vi "decodeStream.vi"(8 "error in (no error)":errorcluster, 9 "beginIndex":i32, 10 "binary stream":u8[](array[numeric]), 11 "tBSONBinary in":refnum<class "tBSONBinary.lvclass">) -> (0 "error out":errorcluster, 1 "endIndex":i32, 2 "binary stream out":u8[](array[numeric]), 3 "tBSONBinary out":refnum<class "tBSONBinary.lvclass">)   [LabVIEW 2013, in "BSON.lvlib" / "tBSONBinary.lvclass"]
uses:
  tBSONBinary.lvclass
  tBSONElement/tBSONElement.lvclass
  status.ctl
  Subtype.ctl
  setSubtype.vi
  setValue.vi
  BSON.lvlib
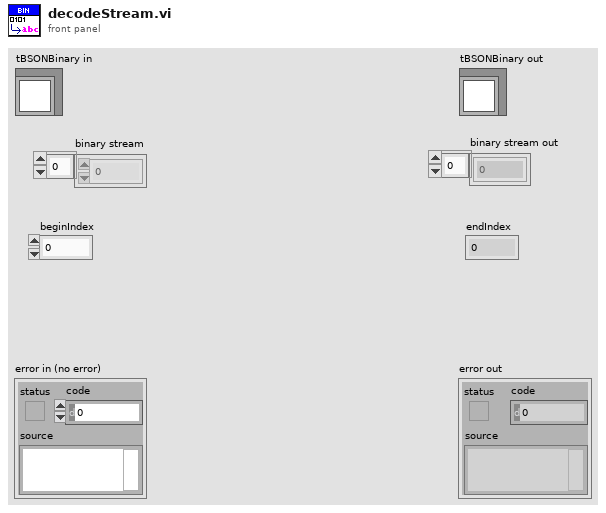
[diagram p1: front panel]
types:
  T1 = typedef "BSON.lvlib/status.ctl" = enum16{"Stream Corrupted or Ended Abruptly", "Incorrect Type In Stream", "ObjectID Invalid", "Method Not Implemented", "Invalid Name", "Invalid URI", "AutoReconnect", "Operation Failed", "Incorrectly Configured", "Cursor Not Found", "Timeout", "Invalid Type", "Empty Name", "Duplicate Name", "MD5Incorrect"}
  T2 = typedef "BSON.lvlib/tBSONBinary.lvclass/Subtype.ctl" = u8
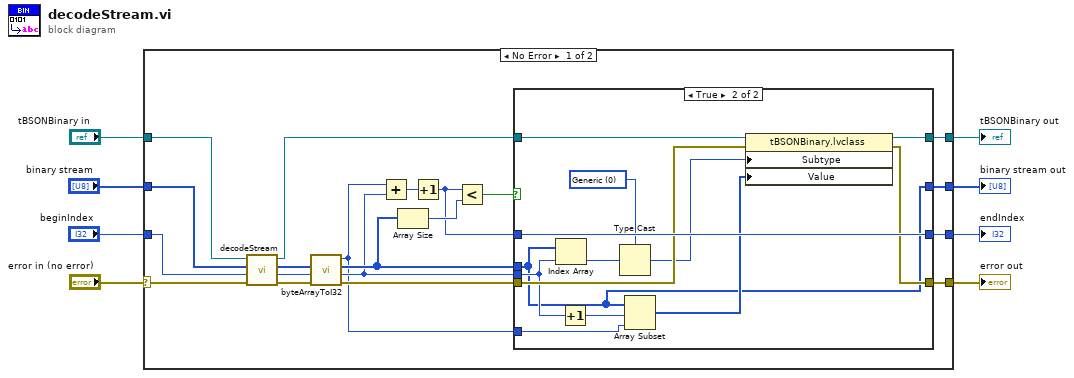
[diagram p0: block diagram]
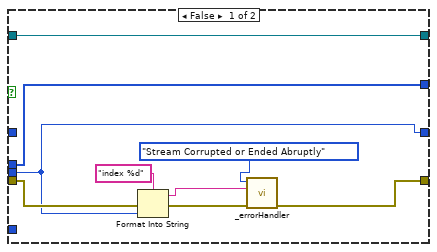
[diagram p2: hidden frame]
diagram:
  n1 = case shown="No Error" "error in (no error)" {
    selector: "error in (no error)" -> [w28 w54]
    tunnel: [w9 w54] -> w7
    tunnel: "beginIndex" -> [w27 w53]
    tunnel: [w17 w53] -> w5
    tunnel: "binary stream" -> [w26 w52]
    tunnel: [w11 w52] -> w3
    tunnel: "tBSONBinary in" -> [w25 w51]
    tunnel: [w12 w51] -> w1
    frame No Error {
      n2 = call-parent "decodeStream.vi"("error in (no error)"=w28, "beginIndex"=w27, "binary stream"=w26, "tBSONElement in"=w25) -> ("error out"=w24:errorcluster, "endIndex"=w22:i32, "binary stream out"=w23:u8[], "tBSONElement out"=w13:refnum<class "tBSONBinary.lvclass">)  [unwired: 4 in]
      n3 = call "byteArrayToI32.vi"("error in (no error)"=w24, "StartIndex"=w22, "ByteArrayIn"=w23) -> ("error out"=w15:errorcluster, "EndIndex"=w14:i32, "ByteArrayOut"=w16:u8[], "I32"=w10:i32)  [unwired: 5 in]
      n4 = Add(x=w10, y=w14) -> (x+y=w21:i32)
      n5 = Array Size(array=w16) -> (size(s)=w20:i32)
      n6 = Increment(x=w21) -> (x+1=w18:i32)
      n7 = Less?(x=w18, y=w20) -> (x < y?=w19:bool)
      n8 = case shown="True" w19 {
        tunnel: w18 -> [_ w50]
        tunnel: [w30 w50] -> w17
        tunnel: w16 -> [w36 w38]
        tunnel: w15 -> [w32 w48]
        tunnel: w14 -> [w30 w42]
        tunnel: w13 -> [w37 w49]
        tunnel: [w37 w47] -> w12
        tunnel: [w36 w38] -> w11
        tunnel: w10 -> [_ w41]
        tunnel: [w31 w39] -> w9
        frame False {
          n9 = Format Into String(format string="index %d", error in=w32, w30) -> (resulting string=w33:string, error out=w34:errorcluster)  [unwired: 1 in]
          n10 = call "_errorHandler.vi"("error in (no error)"=w34, "Additional Text"=w33, "Error Type"=status."Stream Corrupted or Ended Abruptly") -> ("error out"=w31:errorcluster)  [unwired: 8 in]
        }
        frame True {
          w46 = T2 0 items=["Generic"=0, "Function"=1, "Binary (Old)"=2, "UUID"=3, "MD5"=5, "User Defined"=128] ("Type")
          n11 = Index Array(array=w38, index=w42) -> (element=w44:u8)
          n12 = Increment(x=w42) -> (x+1=w43:i32)
          n13 = Type Cast(type=w46, x=w44) -> (*(type *) &x=w45:T2)
          n14 = Array Subset(array=w38, index=w43, length=w41) -> (w40:u8[])
          n15 = property class="tBSONBinary.lvclass"(reference=w49, error in=w48, "Subtype"=w45, "Value"=w40) -> (reference out=w47:refnum<class "tBSONBinary.lvclass">, error out=w39:errorcluster)
        }
      }
    }
    frame Error {
    }
  }
  "error out" <- w7
  "tBSONBinary out" <- w1
  "binary stream out" <- w3
  "endIndex" <- w5
